vi "Find by Path.vi"   [LabVIEW 2015, in "JSONtext.lvlib"]
uses:
  JSONtext.lvlib
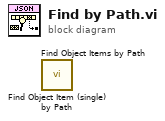
[diagram p0: block diagram]
diagram:
  n1 = call "Find Object Item (single) by Path.vi"() -> ()  [unwired: 8 in, 4 out]
  n2 = call "Find Object Items by Path.vi"() -> ()  [unwired: 8 in, 4 out]
